vi "zero channel physical units.vi"(6 "Index":u32, 7 "Mean (physical units)":dbl format="%.5f") -> ()   [LabVIEW 2012]
uses:
  global scale array.vi
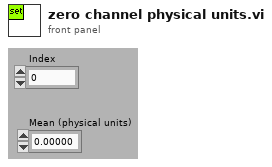
[diagram p1: front panel]
types:
  T1 = typedef "calib array.ctl" = T2[]
  T2 = typedef "conversion.ctl" = cluster{"conversion matrix":sgl[][], "units":string, "name":string, "scale type":T3, "offset (volts)":dbl, "second channel":i8, "correspondence table":T4, "offset (physical units)":dbl, "pH scale":T5, "D.O.":T6}
  T3 = typedef "scale type.ctl" = enum16{"Volts", "Polynomial", "Correspondence Table", "pH", "Dissolved Oxygen", "Quadratic"}
  T4 = typedef "correspondence table.ctl" = cluster{"physical units":dbl, "volts":dbl}[]
  T5 = typedef "pH scale.ctl" = cluster{"Buffers":cluster{"Buffer":dbl, "Calibrated":bool, "V/T":dbl}[], "Temperature":dbl}
  T6 = typedef "DO scale.ctl" = cluster{"Temperature":dbl, "K":dbl, "barometric pressure":dbl}
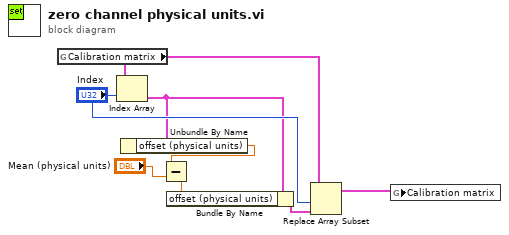
[diagram p0: block diagram]
diagram:
  n1 = global read "global scale array.vi" "Calibration matrix"() -> (w7:T1)
  n2 = Index Array(array=w7, index="Index") -> (element=w4:T2)
  n3 = Unbundle By Name(w4) -> ("offset (physical units)"=w2:dbl)
  n4 = Subtract(x=w2, y="Mean (physical units)") -> (x-y=w3:dbl)
  n5 = Bundle By Name(cluster=w4, "offset (physical units)"=w3) -> (w5:T2)
  n6 = Replace Array Subset(array=w7, new element=w5, index="Index") -> (w6:T1)
  n7 = global write "global scale array.vi" "Calibration matrix"(w6) -> ()
